vi "Module Top Level.vi"(8 "error in":errorcluster) -> (0 "error out":errorcluster)   [LabVIEW 2018, in "PC UDP Writer.lvlib"]
doc: "This is the top level VI for this module. It uses a queue for communications and is stopped user a user event. The general architecture is similar to a simple queued message handler.\n\nThe VIs associated with this module are organized in a LabVIEW Library."
uses:
  PC UDP Writer.lvlib
  Private Controls/cRIO RT Comms Data.ctl
  Top Level/Shared Controls/cRIOData.ctl
  Testing UI 1/Private Controls/APU & ECU Controls.ctl
  Testing UI 1/Public Controls/Bleed-Fuel-ECS Controls.ctl
  Testing UI 3/Private Controls/Cutoff Frequency.ctl
  Private Controls/Module Data.ctl
  Private Controls/Module Action.ctl
  Top Level/Shared Controls/APU Setup File.ctl
  Testing UI 1/Testing UI 1.lvlib
  Testing UI 3/Testing UI 3.lvlib
panel:
  # "UDP Writer"
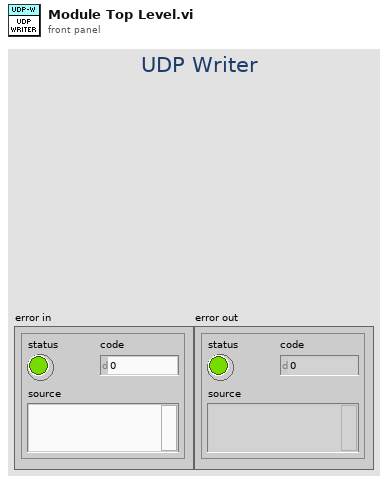
[diagram p1: front panel]
types:
  T1 = typedef "PC UDP Writer.lvlib/cRIO RT Comms Data.ctl" = cluster{"connection ID":refnum<k16>, "cRIO IP":string, "cRIO Port":u16, "cRIO Data":T2}
  T2 = typedef "cRIOData.ctl" = cluster{"APU & ECU Controls":T3, "APU Start":bool, "Bleed Fuel ECS Controls":T4, "FuelPressureReg":dbl, "ECS Demand":dbl, "Accel Sensitivities":dbl[], "Accel Filters":T5[], "ShuntRelay":bool, "Waterfall Select":u8}
  T3 = typedef "Testing UI 1.lvlib/APU & ECU Controls.ctl" = cluster{"02.01.9485.06":bool, "FuelPump":bool, "02.00.9485.01":bool, "02.00.9485.02":bool, "02.00.9485.03":bool, "02.00.9485.05":bool, "02.00.9485.04":bool, "02.00.9485.00":bool, "02.00.9485.07":bool, "02.01.9485.00":bool, "02.01.9485.01":bool}
  T4 = typedef "Testing UI 1.lvlib/Bleed-Fuel-ECS Controls.ctl" = cluster{"Coarse_RC":bool, "Coarse_RO":bool, "Bleed-Fine-Knob":dbl, "Bleed-Coarse-Knob":dbl}
  T5 = typedef "Testing UI 3.lvlib/Cutoff Frequency.ctl" = cluster{"LP Passband":dbl, "HP Stopband":dbl, "LP Stopband":dbl, "HP Passband":dbl}
  T6 = typedef "APU Setup File.ctl" = cluster{"Sensor Info":string[][], "Variables":string[][], "CMM Table 106":string[][], "CMM Table 106B ":string[][], "Accel Config":string[][], "Report Sheet 1":string[][], "Report Sheet 2":string[][], "Report Sheet 3":string[][]}
  T7 = typedef "PC UDP Writer.lvlib/Module Data.ctl" = cluster{"Data":variant, "Action":T8}
  T8 = typedef "PC UDP Writer.lvlib/Module Action.ctl" = enum8{"Init", "Waterfall Select", "Bleed Fuel", "Fuel Pressure Reg", "ECS Demand", "Accel Sensitivities", "Accel Filters", "Shunt Relay", "APU Setup", "APU and ECU Control", "APU Start", "Write", "Error", "Exit"}
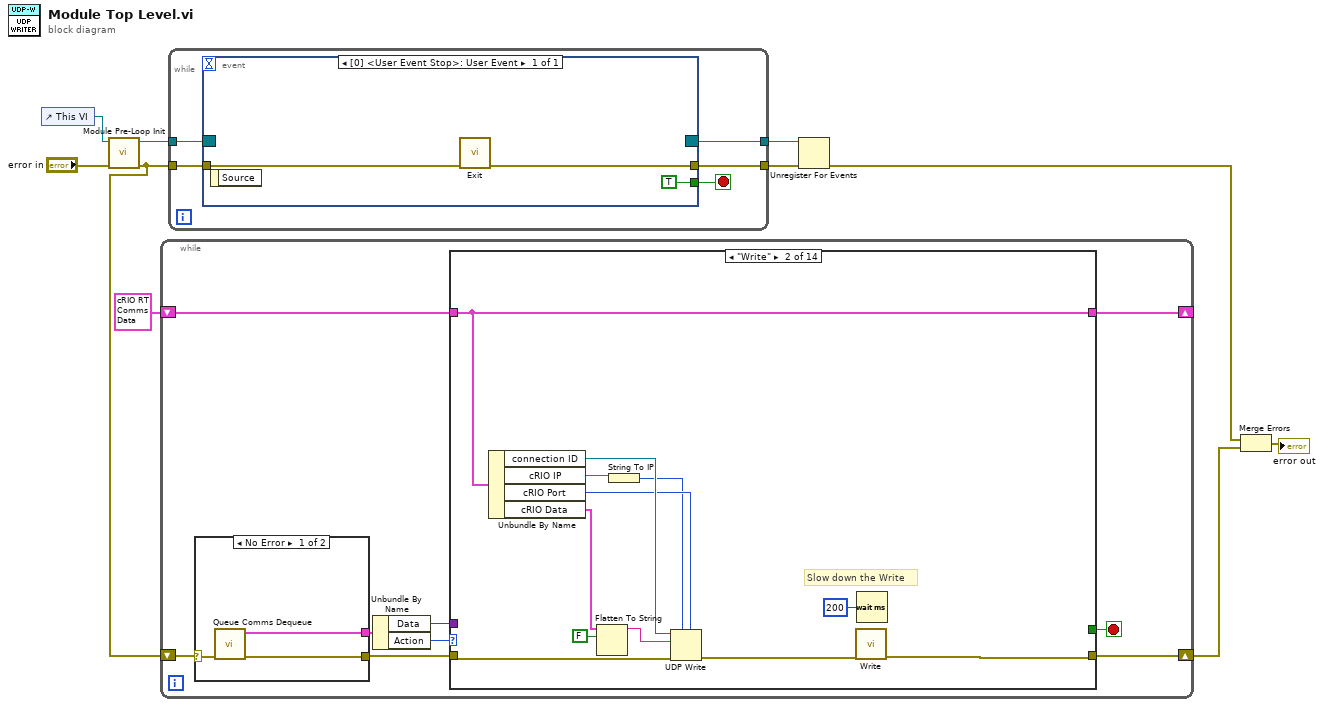
[diagram p0: block diagram]
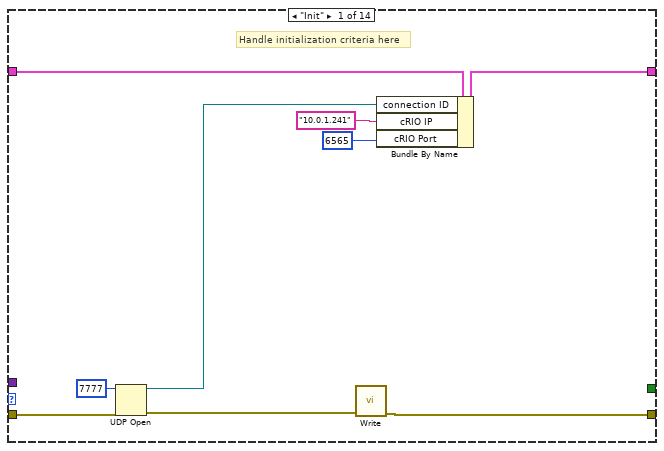
[diagram p2: hidden frame]
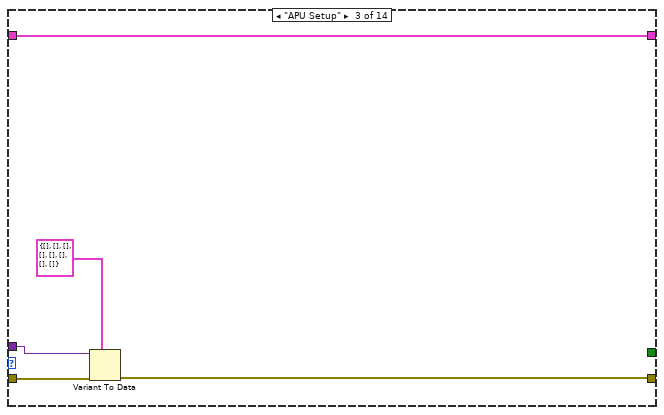
[diagram p3: hidden frame]
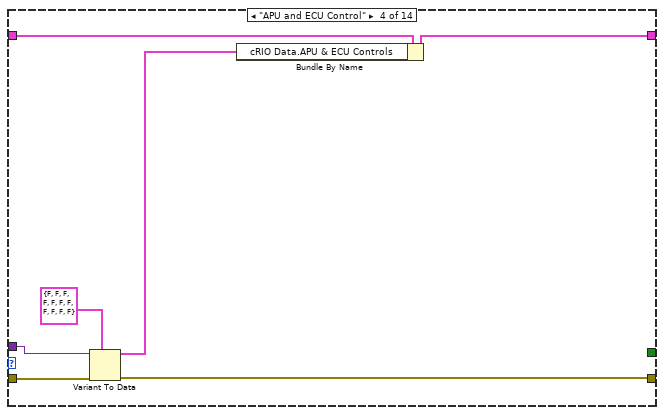
[diagram p4: hidden frame]
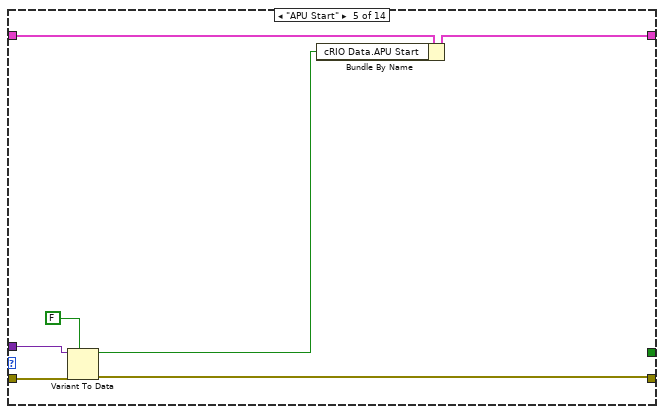
[diagram p5: hidden frame]
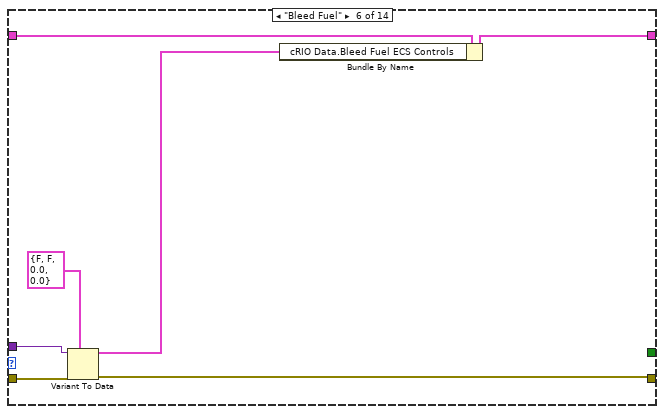
[diagram p6: hidden frame]
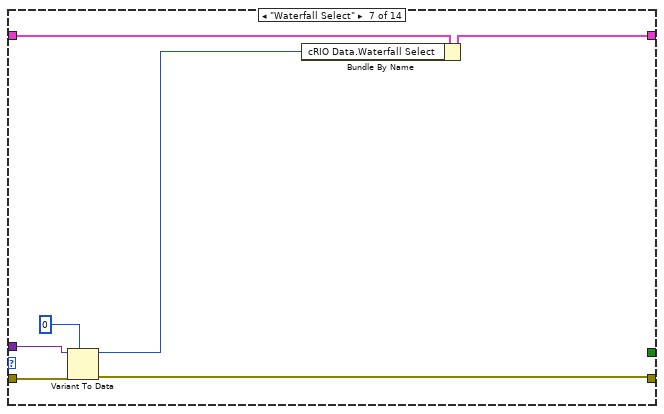
[diagram p7: hidden frame]
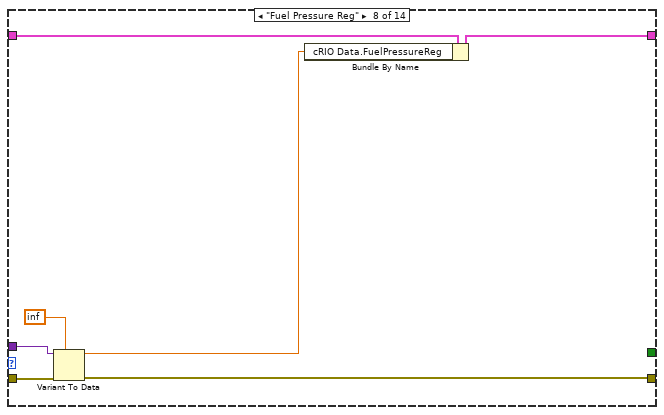
[diagram p8: hidden frame]
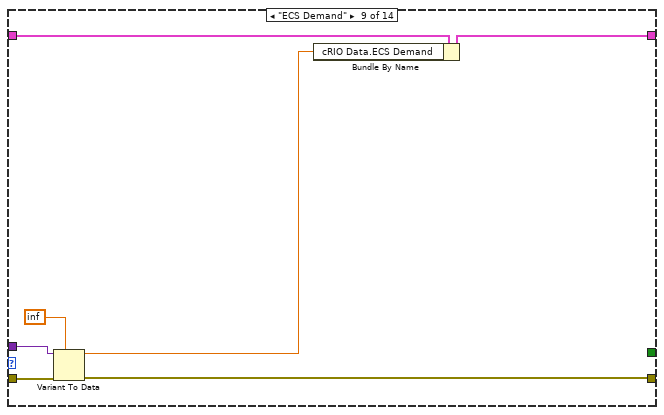
[diagram p9: hidden frame]
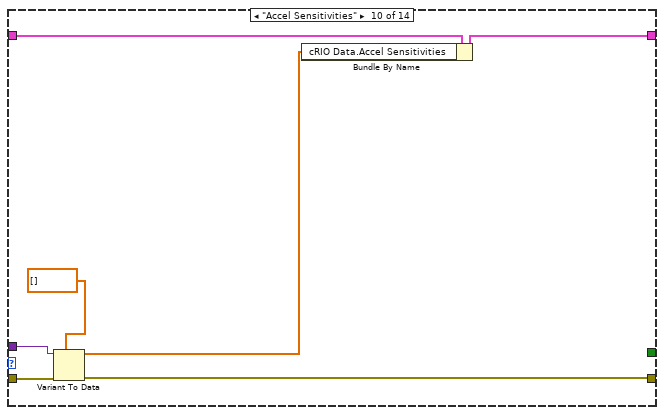
[diagram p10: hidden frame]
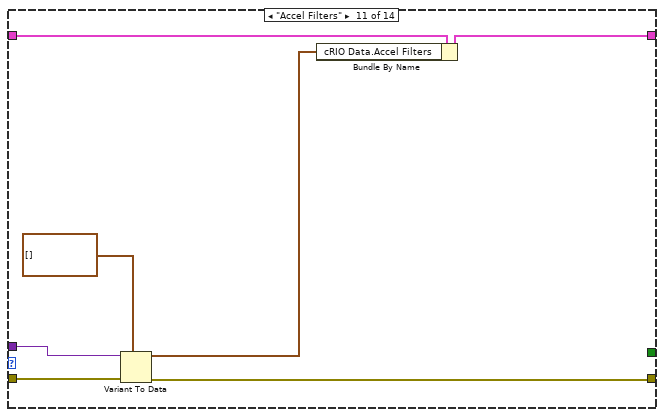
[diagram p11: hidden frame]
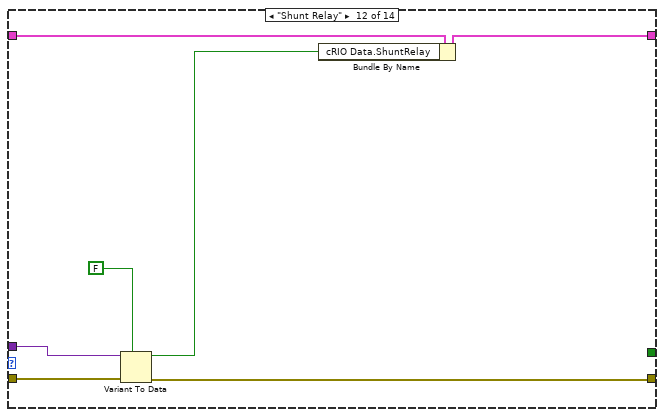
[diagram p12: hidden frame]
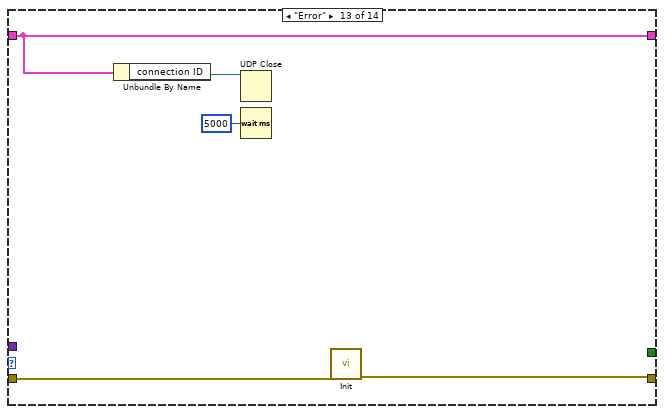
[diagram p13: hidden frame]
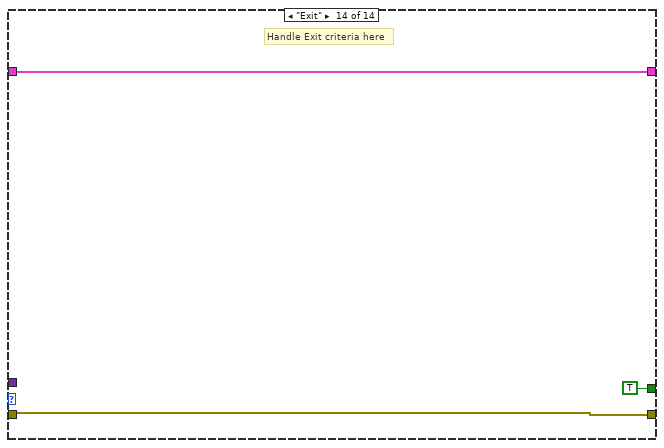
[diagram p14: hidden frame]
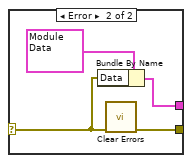
[diagram p15: hidden frame]
diagram:
  n1 = control-ref of="This VI"() -> (w10:refnum<vi>)
  n2 = call "Module Pre-Loop Init.vi"("error in (no error)"="error in", "Top Level VI Ref in"=w10) -> ("error out"=w3:errorcluster, "User Event Stop Ref"=w9:refnum<event-registration>)  [unwired: 8 in]
  n3 = while {
    shift-right: [w14] -> w6
    shift-left: w3 -> [w13]
    shift-right: [w12] -> _
    shift-left: T1 {"connection ID"=refnum, "cRIO IP"="", "cRIO Port"=0, "cRIO Data"={"APU & ECU Controls"={"02.01.9485.06"=FALSE, "FuelPump"=FALSE, "02.00.9485.01"=FALSE, "02.00.9485.02"=FALSE, "02.00.9485.03"=FALSE, "02.00.9485.05"=FALSE, "02.00.9485.04"=FALSE, "02.00.9485.00"=FALSE, "02.00.9485.07"=FALSE, "02.01.9485.00"=FALSE, "02.01.9485.01"=FALSE}, "APU Start"=FALSE, "Bleed Fuel ECS Controls"={"Coarse_RC"=FALSE, "Coarse_RO"=FALSE, "Bleed-Fine-Knob"=0.0, "Bleed-Coarse-Knob"=0.0}, "FuelPressureReg"=0.0, "ECS Demand"=0.0, "Accel Sensitivities"=[], "Accel Filters"=[], "ShuntRelay"=FALSE, "Waterfall Select"=0}} ("cRIO RT Comms Data out") -> [w11]
    stop <- w15 stop-if-true
    n4 = case shown="No Error" w13 {
      selector: w13 -> [w118 w121]
      tunnel: [w119 w122] -> w19
      tunnel: [w117 w120] -> w16
      frame No Error {
        n5 = call "Queue Comms Dequeue.vi"("error in (no error)"=w118) -> ("error out"=w117:errorcluster, "element"=w119:T7)  [unwired: 8 in, 1 out]
      }
      frame Error {
        n6 = Bundle By Name(cluster=T7 {"Data"=variant, "Action"=enum."Error"} ("element"), "Data"=w121) -> (w122:T7)
        n7 = call <vilib>:"Clear Errors.vi"("error in (no error)"=w121) -> ("error out"=w120:errorcluster)  [unwired: 5 in, 1 out]
      }
    }
    n8 = Unbundle By Name(w19) -> ("Data"=w17:variant, "Action"=w18:T8)
    n9 = case shown="\"Write\"" w18 {
      tunnel: w17 -> [_ _ w43 w50 w57 w64 w71 w78 w85 w92 w99 w106 _ _]
      tunnel: w16 -> [w26 w40 w44 w51 w58 w65 w72 w79 w86 w93 w100 w107 w113 w114]
      tunnel: [w20 w33 w41 w47 w55 w63 w70 w74 w81 w89 w96 w103 w110 w114] -> w14
      tunnel: [_ _ _ _ _ _ _ _ _ _ _ _ _ TRUE] -> w15
      tunnel: w11 -> [w28 w39 w45 w52 w59 w66 w73 w80 w87 w94 w101 w108 w112 w115]
      tunnel: [w27 w39 w45 w49 w54 w62 w69 w76 w83 w91 w98 w105 w112 w115] -> w12
      frame "Init" {
        # "Handle initialization criteria here"
        n10 = UDP Open(8:w26, 11:u16 7777 ("port")) -> (port=w24:refnum<k16>, 0:w21:errorcluster)  [unwired: 3 in, 1 out]
        n11 = call "Write.vi"("error in"=w21) -> ("error out"=w20:errorcluster)  [unwired: 10 in]
        n12 = Bundle By Name(cluster=w28, "connection ID"=w24, "cRIO IP"="10.0.1.241", "cRIO Port"=u16 6565) -> (w27:T1)
      }
      frame "Write" {
        # "Slow down the Write"
        n13 = Unbundle By Name(w39) -> ("connection ID"=w38:refnum<k16>, "cRIO IP"=w37:string, "cRIO Port"=w36:u16, "cRIO Data"=w31:T2)
        n14 = Flatten To String(anything=w31, prepend array or string size? (T)=FALSE) -> (data string=w29:string)  [unwired: 2 in, 2 out]
        n15 = String To IP(1:w37) -> (0:w35:u32)
        n16 = UDP Write(address=w35, port or service name=w36, connection ID=w38, data in=w29, 8:w40) -> (error out=w34:errorcluster)  [unwired: 1 in, 1 out]
        n17 = call "Write.vi"("error in"=w34) -> ("error out"=w33:errorcluster)  [unwired: 10 in]
        n18 = Wait (ms)(milliseconds to wait=u32 200) -> ()  [unwired: 1 out]
      }
      frame "APU Setup" {
        n19 = Variant To Data(error in=w44, type=T6 {"Sensor Info"=[], "Variables"=[], "CMM Table 106"=[], "CMM Table 106B "=[], "Accel Config"=[], "Report Sheet 1"=[], "Report Sheet 2"=[], "Report Sheet 3"=[]} ("APU Setup File"), Variant=w43) -> (error out=w41:errorcluster)  [unwired: 1 out]
      }
      frame "APU and ECU Control" {
        n20 = Variant To Data(error in=w51, type=T3 {"02.01.9485.06"=FALSE, "FuelPump"=FALSE, "02.00.9485.01"=FALSE, "02.00.9485.02"=FALSE, "02.00.9485.03"=FALSE, "02.00.9485.05"=FALSE, "02.00.9485.04"=FALSE, "02.00.9485.00"=FALSE, "02.00.9485.07"=FALSE, "02.01.9485.00"=FALSE, "02.01.9485.01"=FALSE} ("output cluster"), Variant=w50) -> (data=w48:T3, error out=w47:errorcluster)
        n21 = Bundle By Name(cluster=w52, "cRIO Data.APU & ECU Controls"=w48) -> (w49:T1)
      }
      frame "APU Start" {
        n22 = Variant To Data(error in=w58, type=FALSE, Variant=w57) -> (data=w53:bool, error out=w55:errorcluster)
        n23 = Bundle By Name(cluster=w59, "cRIO Data.APU Start"=w53) -> (w54:T1)
      }
      frame "Bleed Fuel" {
        n24 = Variant To Data(error in=w65, type=T4 {"Coarse_RC"=FALSE, "Coarse_RO"=FALSE, "Bleed-Fine-Knob"=0.0, "Bleed-Coarse-Knob"=0.0} ("Bleed Fuel ECS Controls"), Variant=w64) -> (data=w61:T4, error out=w63:errorcluster)
        n25 = Bundle By Name(cluster=w66, "cRIO Data.Bleed Fuel ECS Controls"=w61) -> (w62:T1)
      }
      frame "Waterfall Select" {
        n26 = Variant To Data(error in=w72, type=u8 0, Variant=w71) -> (data=w68:u8, error out=w70:errorcluster)
        n27 = Bundle By Name(cluster=w73, "cRIO Data.Waterfall Select"=w68) -> (w69:T1)
      }
      frame "Fuel Pressure Reg" {
        n28 = Variant To Data(error in=w79, type=inf, Variant=w78) -> (data=w75:dbl, error out=w74:errorcluster)
        n29 = Bundle By Name(cluster=w80, "cRIO Data.FuelPressureReg"=w75) -> (w76:T1)
      }
      frame "ECS Demand" {
        n30 = Variant To Data(error in=w86, type=inf, Variant=w85) -> (data=w82:dbl, error out=w81:errorcluster)
        n31 = Bundle By Name(cluster=w87, "cRIO Data.ECS Demand"=w82) -> (w83:T1)
      }
      frame "Accel Sensitivities" {
        n32 = Variant To Data(error in=w93, type=dbl[] [] ("appended array"), Variant=w92) -> (data=w90:dbl[], error out=w89:errorcluster)
        n33 = Bundle By Name(cluster=w94, "cRIO Data.Accel Sensitivities"=w90) -> (w91:T1)
      }
      frame "Accel Filters" {
        n34 = Variant To Data(error in=w100, type=T5[] [] ("Cutoff Frequency"), Variant=w99) -> (data=w97:T5[], error out=w96:errorcluster)
        n35 = Bundle By Name(cluster=w101, "cRIO Data.Accel Filters"=w97) -> (w98:T1)
      }
      frame "Shunt Relay" {
        n36 = Variant To Data(error in=w107, type=FALSE, Variant=w106) -> (data=w104:bool, error out=w103:errorcluster)
        n37 = Bundle By Name(cluster=w108, "cRIO Data.ShuntRelay"=w104) -> (w105:T1)
      }
      frame "Error" {
        n38 = Unbundle By Name(w112) -> ("connection ID"=w111:refnum<k16>)
        n39 = UDP Close(connection ID=w111) -> ()  [unwired: 1 in, 2 out]
        n40 = Wait (ms)(milliseconds to wait=u32 5000) -> ()  [unwired: 1 out]
        n41 = call "Init.vi"("error in"=w113) -> ("error out"=w110:errorcluster)  [unwired: 10 in]
      }
      frame "Exit" {
        # "Handle Exit criteria here"
      }
    }
  }
  n42 = while {
    tunnel: w9 -> [w128]
    tunnel: [w127] -> w7
    tunnel: w3 -> [w126]
    tunnel: [w124] -> w8
    stop <- w125 stop-if-true
    n43 = event shown="[0] <User Event Stop>: User Event" {
      selector: w128 -> [_]
      dyn-events: [_] -> w124
      timeout: _ -> [_]
      tunnel: [w129] -> w127
      tunnel: w126 -> [w130]
      tunnel: [TRUE] -> w125
      event User Event {
        n44 = event-data() -> ()  [unwired: 1 in, 1 out]
        n45 = call "Exit.vi"("error in (no error)"=w130) -> ("error out"=w129:errorcluster)  [unwired: 10 in]
      }
    }
  }
  n46 = Unregister For Events(event registration refnum=w8, error in=w7) -> (error out=w5:errorcluster)
  n47 = Merge Errors(w5, w6) -> (→"error out":errorcluster)
